vi "NIIE_Fire Body Text Change event.vi"(8 "error in":errorcluster, 11 "Ref.Body Text":refnum<vi>) -> (0 "error out":errorcluster)   [LabVIEW 2021]
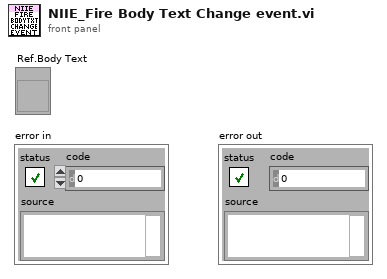
[diagram p1: front panel]
types:
  T1 = typedef "Font.ctl" = string
  T2 = typedef "Alignment.ctl" = u16
  T3 = typedef "Font Size.ctl" = u8
  T4 = cluster{"Line 1 text":string, "Line 2 text":string, "Line 3 text":string, "Line 4 text":string, "Line 1 color":u32, "Line 2 color":u32, "Line 3 color":u32, "Line 4 color":u32, "Body Text Spec":cluster{"DNL_Font":T1, "Alignment":T2, "Size":T3}, "Center text vertically":bool, "Capitalize Text":bool}
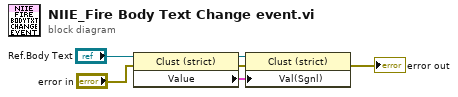
[diagram p0: block diagram]
diagram:
  n1 = property class="Clust (strict)"(reference="Ref.Body Text", error in="error in") -> (reference out=w2:refnum<vi>, error out=w3:errorcluster, "Value"=w4:T4)
  n2 = property class="Clust (strict)"(reference=w2, error in=w3, "Val(Sgnl)"=w4) -> (error out=→"error out":errorcluster)  [unwired: 1 out]
